vi "Agilent 34970 Get Data Main.vi"(8 "error in (no error)":errorcluster, 10 "Analog Channels-List":string, 11 "VISA Refnum in":refnum<visa-resource-name>) -> (0 "error out":errorcluster, 1 "read buffer":string, 2 "Sorted Data":dbl[](array[numeric]), 3 "VISA Resource Name Out":refnum<visa-resource-name>, 4 "Names":string[](array[string]), 6 "UnSorted Data":dbl[](array[numeric]) format="%.2f")   [LabVIEW 2020]
uses:
  Agilent 34970.lvlib
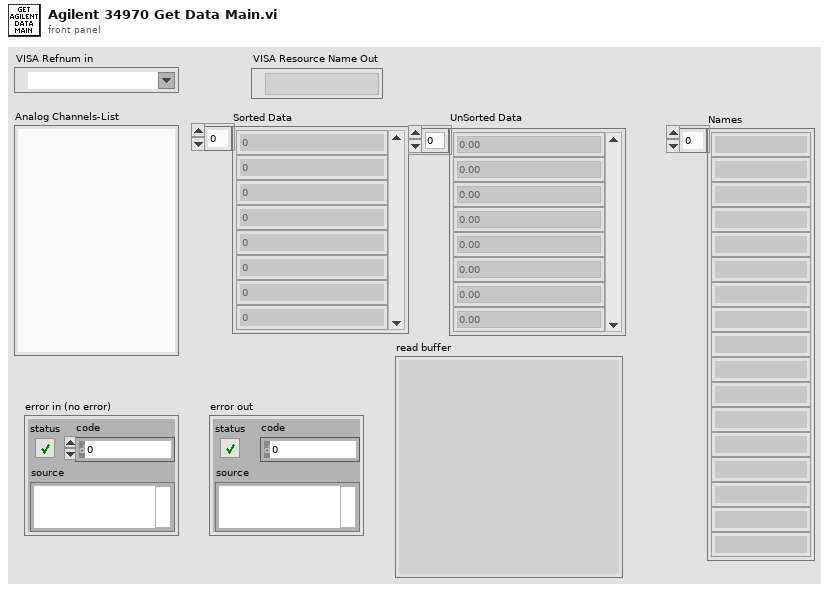
[diagram p1: front panel]
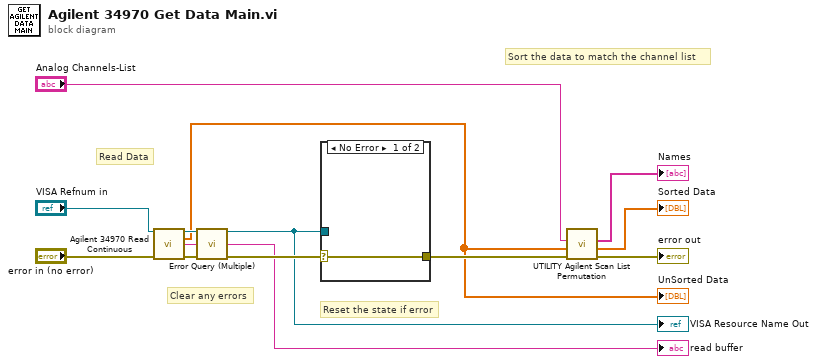
[diagram p0: block diagram]
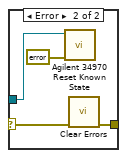
[diagram p2: hidden frame]
diagram:
  # "Sort the data to match the channel list"
  # "Reset the state if error"
  # "Clear any errors"
  # "Read Data"
  n1 = call "Agilent 34970 Read Continuous.vi"("VISA Resource Name"="VISA Refnum in", "error in (no error)"="error in (no error)") -> ("VISA resource name out"=w11:refnum<visa-resource-name>, "Output Array"=w5:dbl[], "read buffer"=→"read buffer":string, "error out"=w10:errorcluster)  [unwired: 10 in]
  "UnSorted Data" <- w5
  n2 = call "Error Query (Multiple).vi"("VISA Resource Name"=w11, "error in (no error)"=w10) -> ("VISA Resource Name Out"=w12:refnum<visa-resource-name>, "error out"=w13:errorcluster)  [unwired: 10 in, 2 out]
  "VISA Resource Name Out" <- w12
  n3 = case shown="No Error" w13 {
    selector: w13 -> [w14 w16]
    tunnel: [w14 w15] -> w9
    tunnel: w12 -> [_ w18]
    frame No Error {
    }
    frame Error {
      n4 = call "Agilent 34970 Reset Known State.vi"("Error In"=errorcluster {"status"=TRUE, "code"=0, "source"=""}, "VISA Refnum in"=w18) -> ()  [unwired: 9 in, 1 out]
      n5 = call <vilib>:"Clear Errors.vi"("error in (no error)"=w16) -> ("error out"=w15:errorcluster)  [unwired: 5 in, 1 out]
    }
  }
  n6 = call "UTILITY Agilent Scan List Permutation.vi"("Error In"=w9, "Input Data Array"=w5, "Agilent Scan List"="Analog Channels-List") -> ("Error Out"=→"error out":errorcluster, "Output Data Permutation"=→"Sorted Data":dbl[], "Names"=→"Names":string[])  [unwired: 6 in]
